vi "AlexMonitoring.vi"(8 "alexRight/Buttons":bool[](array[boolean]), 9 "alexRight/Axes":dbl[](array[numeric]), 10 "alexLeft/Buttons":bool[](array[boolean]), 11 "alexLeft/Axes":dbl[](array[numeric])) -> ()   [LabVIEW 2012]
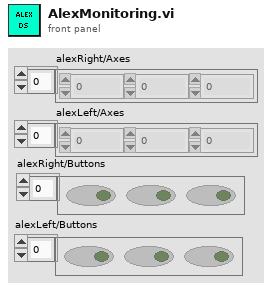
[diagram p1: front panel]
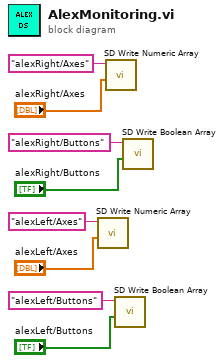
[diagram p0: block diagram]
diagram:
  n1 = call <vilib>:"SD Write Numeric Array.vi"("Numeric Array"="alexLeft/Axes", "Name"="alexLeft/Axes") -> ()  [unwired: 8 in, 2 out]
  n2 = call <vilib>:"SD Write Numeric Array.vi"("Numeric Array"="alexRight/Axes", "Name"="alexRight/Axes") -> ()  [unwired: 8 in, 2 out]
  n3 = call <vilib>:"SD Write Boolean Array.vi"("Boolean Array"="alexLeft/Buttons", "Name"="alexLeft/Buttons") -> ()  [unwired: 8 in, 2 out]
  n4 = call <vilib>:"SD Write Boolean Array.vi"("Boolean Array"="alexRight/Buttons", "Name"="alexRight/Buttons") -> ()  [unwired: 8 in, 2 out]
